vi "SignalThreshold.vi"(0 "Signal in":waveform(dbl), 1 "Low cutoff freq (Hz)":dbl, 2 "High cutoff freq (Hz)":dbl, 5 "Audio sample rate (Hz)":i64, 7 "High threshold (Vrms)":dbl=0.1, 9 "Low threshold (Vrms)":dbl=0.1) -> (4 "Filtered signal":waveform(dbl), 6 "Mean above high threshold?":bool, 8 "Mean below low threshold?":bool, 10 "Amplitude":dbl format="%0.2f")   [LabVIEW 2017]
doc: "Take in an audio signal, bandpass filter it, measure the mean RMS amplitude for a high\nand low monitoring period"
uses:
  <vilib>/Analysis/3filter.llb/Filter Passband Type.ctl
  <vilib>/Analysis/baseanly.llb/Mean (DBL).vi
  <vilib>/Analysis/5stat.llb/RMS (DBL).vi
  <vilib>/Analysis/3filter.llb/Butterworth Filter (DBL).vi
  <vilib>/Analysis/NI_AALBase.lvlib
  <vilib>/Analysis/NI_AALPro.lvlib
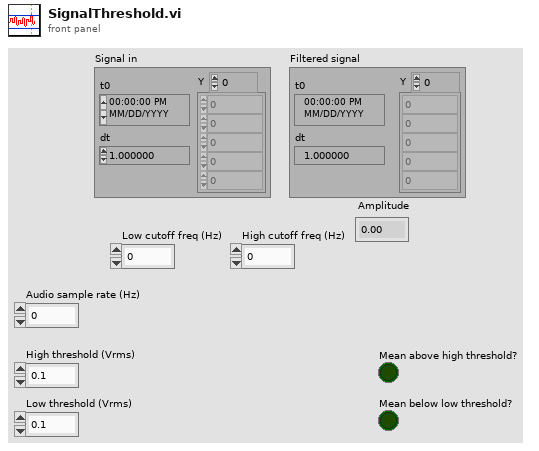
[diagram p1: front panel]
types:
  T1 = typedef "NI_AALBase.lvlib/Filter Passband Type.ctl" = enum32{"Lowpass", "Highpass", "Bandpass", "Bandstop"}
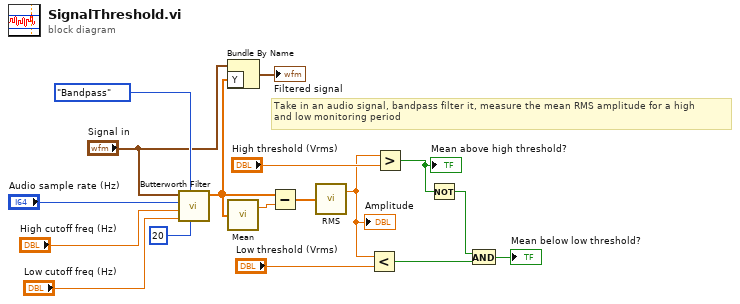
[diagram p0: block diagram]
diagram:
  # "Take in an audio signal, bandpass filter it, measure the mean RMS amplitude for a high\nand low monitoring period"
  n1 = call-poly <vilib>:"Butterworth Filter.vi"("order"=20, "filter type"=Filter_Passband_Type."Bandpass", "low cutoff freq: fl"="Low cutoff freq (Hz)", "high cutoff freq: fh"="High cutoff freq (Hz)", "sampling freq: fs"="Audio sample rate (Hz)", "X"="Signal in") -> ("Filtered X"=w3:dbl[])  [unwired: 2 in, 1 out]
  n2 = Bundle By Name(cluster="Signal in", "Y"=w3) -> (→"Filtered signal":waveform(dbl))
  n3 = call-poly <vilib>:"Mean.vi"("X"=w3) -> ("mean"=w11:dbl)  [unwired: 1 out]
  n4 = Subtract(x=w3, y=w11) -> (x-y=w4:dbl[])
  n5 = call-poly <vilib>:"RMS.vi"("X"=w4) -> ("rms value"=w2:dbl)  [unwired: 1 out]
  "Amplitude" <- w2
  n6 = Less?(x=w2, y="Low threshold (Vrms)") -> (x < y?=w7:bool)
  n7 = Greater?(x=w2, y="High threshold (Vrms)") -> (0:w9:bool)
  "Mean above high threshold?" <- w9
  n8 = Not(x=w9) -> (.not. x?=w15:bool)
  n9 = And(x=w15, y=w7) -> (x .and. y?=→"Mean below low threshold?":bool)
